vi "Connect to ACCDB Database.vi"() -> ()   [LabVIEW 2023]
doc: "This example demonstrates how to read data from a Microsoft Access 2007 database file. You must use the ACE engine instead of the JET engine to access the database. The example database file, Access2007.accdb, is located in the labview\\examples\\database directory.\n\nRun this VI to display all the data from the example ACCDB database. Examine the block diagram of this VI to see how to use the Database Variant To Data function to convert a database variant to the data type you need."
uses:
  <vilib>/addons/database/Connection.llb/DB Tools Open Connec (String).vi
  <vilib>/addons/database/_DB Variant To Data/Database Variant To Data.xnode
  <vilib>/addons/database/NI_Database_API.lvlib
panel:
  out "Data returned from ACCDB file":cluster{"String":string, "I32":i32, "DBL":dbl}[](array[cluster])
  # "Overview: Demonstrates how to read data from a Microsoft Access 2007 database file.\nRequirements: Database Connectivity Toolkit, Office System Driver: Data Connectivity Components version 2007 or later\nInstructions:\nRun the VI to display all the data from the example ACCDB database. If an error occurs, you may need to install the Office System Driver: Data Connectivity Components version 2007 or later."
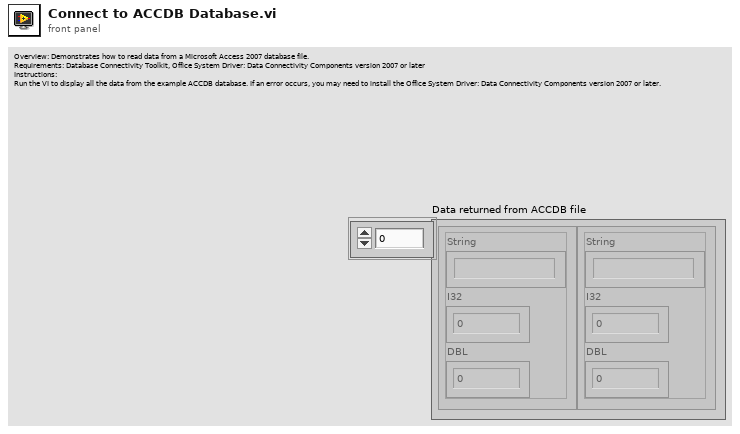
[diagram p1: front panel]
types:
  T1 = typedef "NI_Database_API.lvlib/Conn ObjectReference.ctl" = refnum<k1>
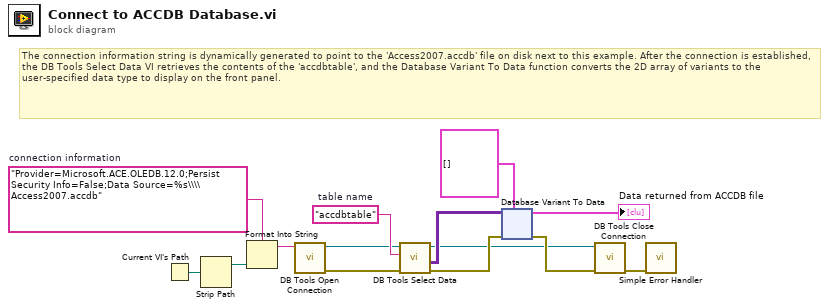
[diagram p0: block diagram]
diagram:
  w2 = "Provider=Microsoft.ACE.OLEDB.12.0;Persist Security Info=False;Data Source=%s\\\\Access2007.accdb"  # connection information
  w14 = "accdbtable"  # table name
  # "The connection information string is dynamically generated to point to the 'Access2007.accdb' file on disk next to this example. After the connection is established, the DB Tools Select Data VI retrieves the contents of the 'accdbtable', and the Database Variant To Data function converts the 2D array of variants to the user-specified data type to display on the front panel."
  n1 = Current VI's Path() -> (path=w7:path)
  n2 = Strip Path(path=w7) -> (stripped path=w3:path)  [unwired: 1 out]
  n3 = Format Into String(format string=w2, w3) -> (resulting string=w4:string)  [unwired: 2 in, 1 out]
  n4 = call-poly <vilib>:"DB Tools Open Connection.vi"("connection information"=w4) -> ("error out"=w12:errorcluster, "connection reference"=w13:T1)  [unwired: 7 in]
  n5 = call <vilib>:"DB Tools Select Data.vi"("error in (no error)"=w12, "table"=w14, "connection reference"=w13) -> ("error out"=w11:errorcluster, "data"=w9:variant[][], "connection reference out"=w8:T1)  [unwired: 3 in]
  n6 = xnode "Database Variant To Data"("database variant"=w9, "error in (no error)"=w11, "type"=cluster{string, i32, dbl}[] []) -> ("data"=→"Data returned from ACCDB file":cluster{string, i32, dbl}[], "error out"=w10:errorcluster)
  n7 = call <vilib>:"DB Tools Close Connection.vi"("error in (no error)"=w10, "connection reference"=w8) -> ("error out"=w6:errorcluster)  [unwired: 5 in]
  n8 = call <vilib>:"Simple Error Handler.vi"("error in (no error)"=w6) -> ()  [unwired: 4 in, 5 out]
